vi "Lab 1.vi"() -> ()   [LabVIEW 2016]
panel:
  in  "quarter":bool
  in  "dime":bool
  in  "nickel":bool
  in  "while loop":bool
  in  "TAKE SODA":bool
  out "you get a coke!":bool
  out "coins returned":dbl
  out "amount inserted":dbl
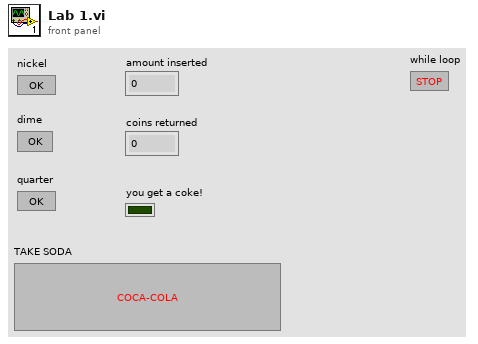
[diagram p1: front panel]
types:
  T1 = enum16{"Init", "5 Cents", "10 Cents", "15 Cents", "20 Cents", "25 Cents", "30 Cents", "35 Cents", "40 Cents", "45 Cents"}
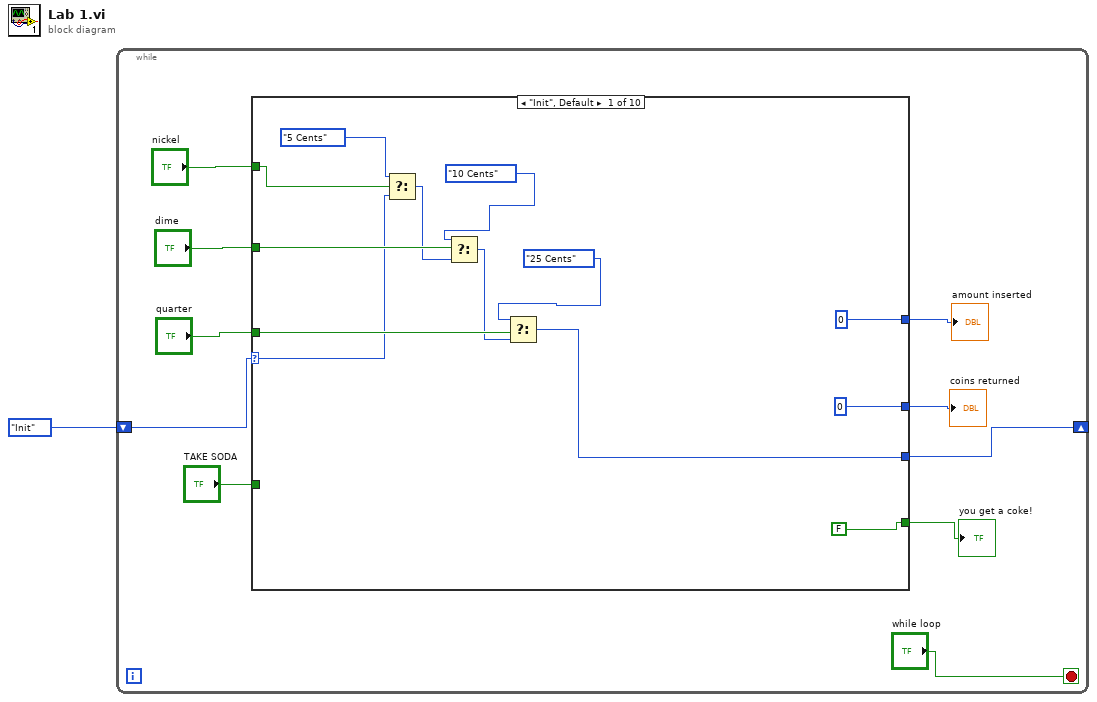
[diagram p0: block diagram]
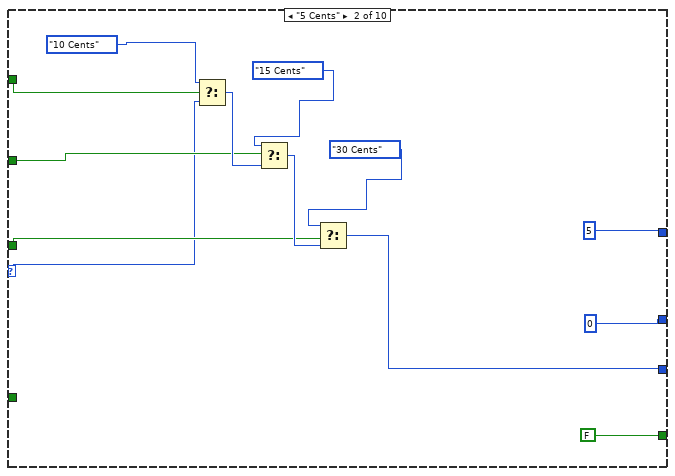
[diagram p2: hidden frame]
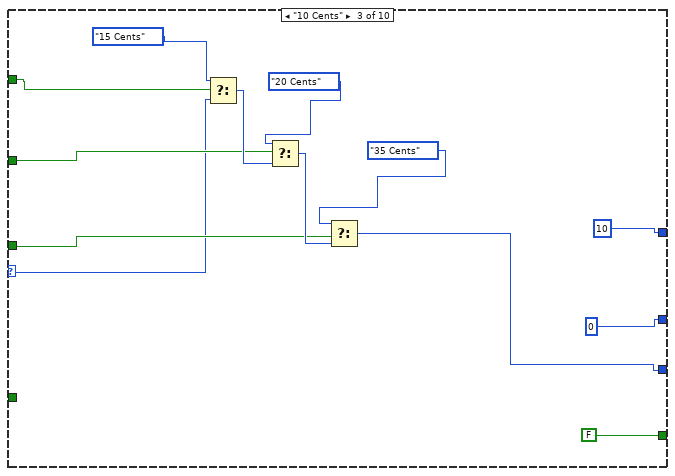
[diagram p3: hidden frame]
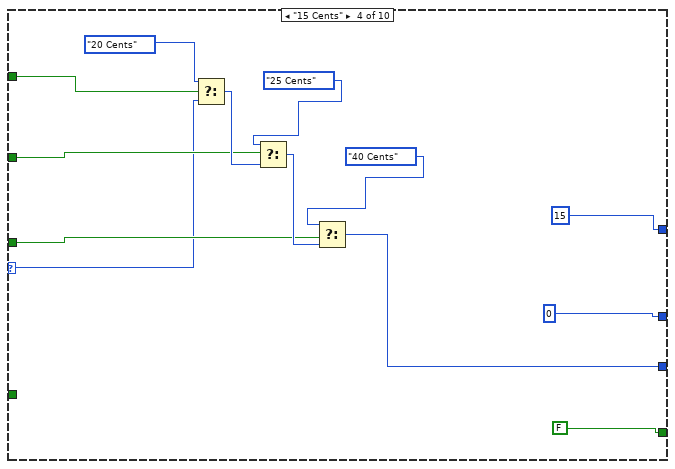
[diagram p4: hidden frame]
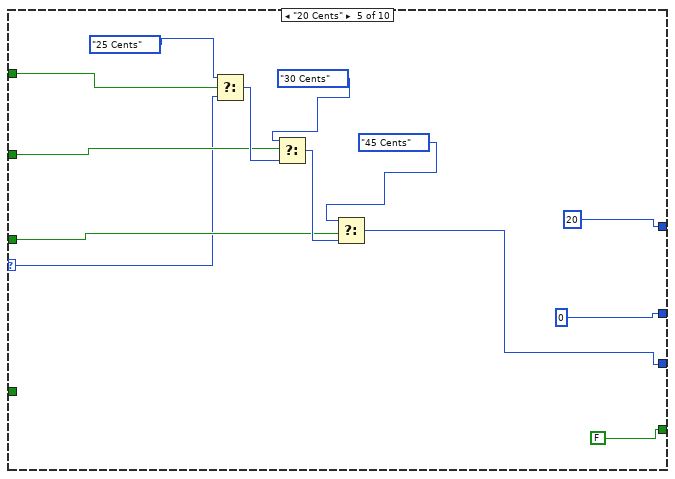
[diagram p5: hidden frame]
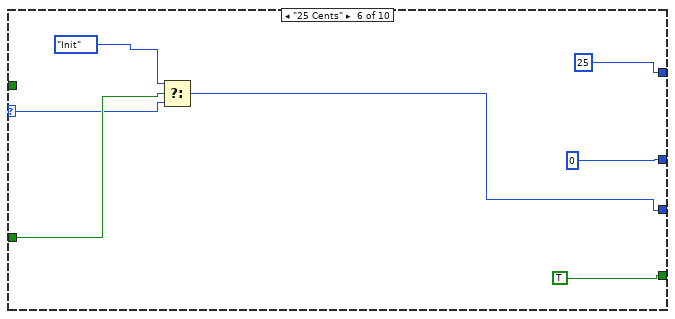
[diagram p6: hidden frame]
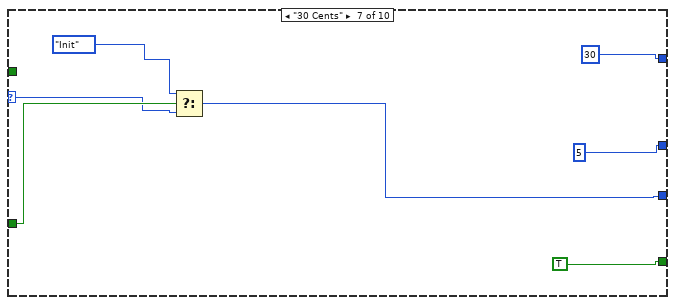
[diagram p7: hidden frame]
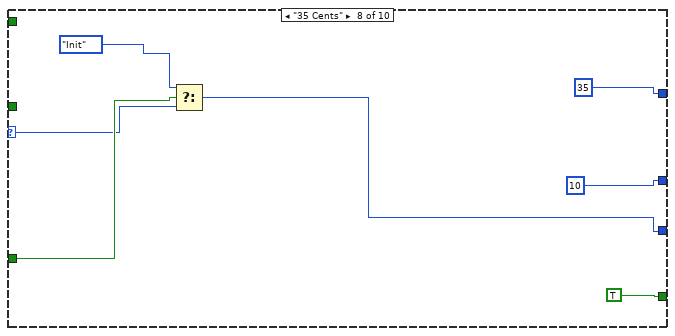
[diagram p8: hidden frame]
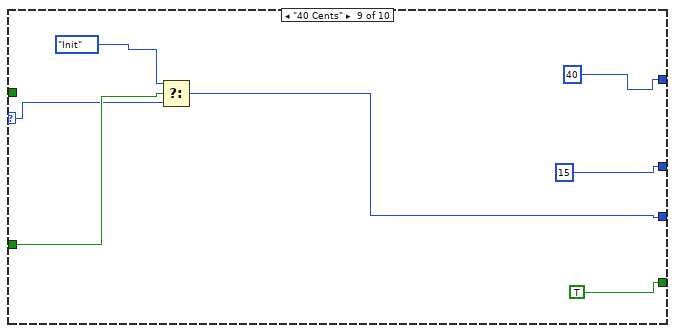
[diagram p9: hidden frame]
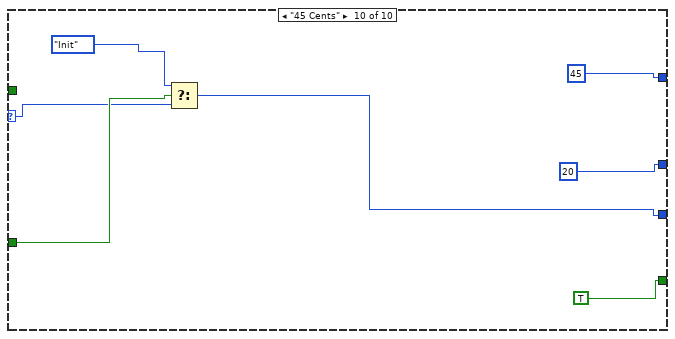
[diagram p10: hidden frame]
diagram:
  n1 = while {
    shift-right: [w7] -> _
    shift-left: T1."Init" -> [w8]
    stop <- "while loop" stop-if-true
    n2 = case shown="\"Init\", Default" w8 {
      selector: w8 -> [w18 w29 w42 w55 w68 w79 w86 w93 w100 w107]
      tunnel: [0 5 10 15 20 25 30 35 40 45] -> w11
      tunnel: [0 0 0 0 0 0 5 10 15 20] -> w10
      tunnel: [FALSE FALSE FALSE FALSE FALSE TRUE TRUE TRUE TRUE TRUE] -> w9
      tunnel: "nickel" -> [w21 w32 w45 w58 w71 _ _ _ _ _]
      tunnel: "dime" -> [w20 w31 w44 w57 w70 _ _ _ _ _]
      tunnel: "quarter" -> [w19 w30 w43 w56 w69 _ _ _ _ _]
      tunnel: [w15 w28 w41 w54 w67 w78 w85 w92 w99 w106] -> w7
      tunnel: "TAKE SODA" -> [_ _ _ _ _ w80 w87 w94 w101 w108]
      frame "Init", Default {
        n3 = Select(t=T1."5 Cents", s=w21, f=w18) -> (s? t:f=w17:T1)
        n4 = Select(t=T1."10 Cents", s=w20, f=w17) -> (s? t:f=w16:T1)
        n5 = Select(t=T1."25 Cents", s=w19, f=w16) -> (s? t:f=w15:T1)
      }
      frame "5 Cents" {
        n6 = Select(t=T1."10 Cents", s=w32, f=w29) -> (s? t:f=w33:T1)
        n7 = Select(t=T1."15 Cents", s=w31, f=w33) -> (s? t:f=w34:T1)
        n8 = Select(t=T1."30 Cents", s=w30, f=w34) -> (s? t:f=w28:T1)
      }
      frame "10 Cents" {
        n9 = Select(t=T1."15 Cents", s=w45, f=w42) -> (s? t:f=w47:T1)
        n10 = Select(t=T1."20 Cents", s=w44, f=w47) -> (s? t:f=w46:T1)
        n11 = Select(t=T1."35 Cents", s=w43, f=w46) -> (s? t:f=w41:T1)
      }
      frame "15 Cents" {
        n12 = Select(t=T1."20 Cents", s=w58, f=w55) -> (s? t:f=w59:T1)
        n13 = Select(t=T1."25 Cents", s=w57, f=w59) -> (s? t:f=w60:T1)
        n14 = Select(t=T1."40 Cents", s=w56, f=w60) -> (s? t:f=w54:T1)
      }
      frame "20 Cents" {
        n15 = Select(t=T1."25 Cents", s=w71, f=w68) -> (s? t:f=w72:T1)
        n16 = Select(t=T1."30 Cents", s=w70, f=w72) -> (s? t:f=w73:T1)
        n17 = Select(t=T1."45 Cents", s=w69, f=w73) -> (s? t:f=w67:T1)
      }
      frame "25 Cents" {
        n18 = Select(t=T1."Init", s=w80, f=w79) -> (s? t:f=w78:T1)
      }
      frame "30 Cents" {
        n19 = Select(t=T1."Init", s=w87, f=w86) -> (s? t:f=w85:T1)
      }
      frame "35 Cents" {
        n20 = Select(t=T1."Init", s=w94, f=w93) -> (s? t:f=w92:T1)
      }
      frame "40 Cents" {
        n21 = Select(t=T1."Init", s=w101, f=w100) -> (s? t:f=w99:T1)
      }
      frame "45 Cents" {
        n22 = Select(t=T1."Init", s=w108, f=w107) -> (s? t:f=w106:T1)
      }
    }
    "amount inserted" <- w11
    "coins returned" <- w10
    "you get a coke!" <- w9
  }
